vi "Plot Helper.vi"   [LabVIEW 2017, in "3D Quiver Datatype.lvclass"]
doc: "Graphs a plot of normal vectors. Multiple references to this VI generate multiple plots for the same graph."
uses:
  <vilib>/Math Plots/3D Math Plots/3D Quiver/3D Quiver Datatype/3D Quiver Datatype.lvclass
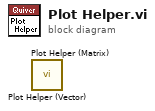
[diagram p0: block diagram]
diagram:
  n1 = call <vilib>:"Plot Helper (Vector).vi"() -> ()  [unwired: 14 in, 2 out]
  n2 = call <vilib>:"Plot Helper (Matrix).vi"() -> ()  [unwired: 14 in, 2 out]
